vi "Delete Variable Handle.vi"(8 "error in (no error)":errorcluster, 10 "Handle":i32, 11 "TwinCAT ADS in":refnum<class "TwinCAT ADS.lvclass">) -> (0 "error out":errorcluster, 3 "TwinCAT ADS out":refnum<class "TwinCAT ADS.lvclass">)   [LabVIEW 2018, in "TwinCAT ADS.lvclass"]
uses:
  TwinCAT ADS.lvclass
  TwinCAT ADS.lvclass/TwinCAT ADS.ctl
  TwinCAT.Ads
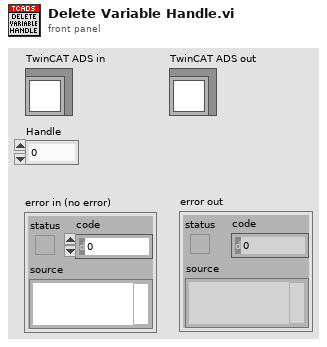
[diagram p1: front panel]
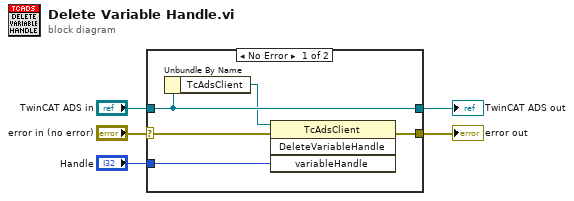
[diagram p0: block diagram]
diagram:
  n1 = case shown="No Error" "error in (no error)" {
    selector: "error in (no error)" -> [w9 w12]
    tunnel: [w6 w12] -> w4
    tunnel: [w10 w11] -> w2
    tunnel: "TwinCAT ADS in" -> [w10 w11]
    tunnel: "Handle" -> [w7 _]
    frame No Error {
      n2 = Unbundle By Name(w10) -> ("TcAdsClient"=w8:refnum<k24>)
      n3 = invoke class="TcAdsClient" method="DeleteVariableHandle"(reference=w8, error in=w9, "variableHandle"=w7) -> (error out=w6:errorcluster)  [unwired: 1 in, 3 out]
    }
    frame Error {
    }
  }
  "error out" <- w4
  "TwinCAT ADS out" <- w2
